vi "Sensor Indicator Map.vi"(8 "Action":T1, 10 "Control Lists In":refnum<vi>[][](array[refnum]), 11 "Sensor List In":T2[](array[typedef])) -> (2 "Control Lists Out":refnum<vi>[][](array[refnum]), 3 "Sensor List Out":T2[](array[typedef]))   [LabVIEW 2015]
uses:
  Sensor Enum.ctl
  Sensor Indicator Map Action.ctl
panel:
  in  "Sensor Enum":T2
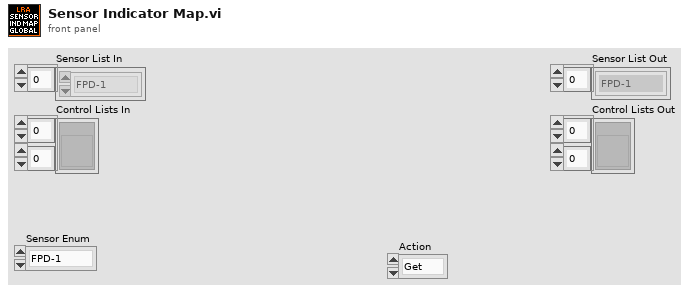
[diagram p1: front panel]
types:
  T1 = typedef "Sensor Indicator Map Action.ctl" = enum16{"Get", "Set"}
  T2 = typedef "Sensor Enum.ctl" = enum16{"FPD-1", "FPD-2", "FPD-3", "OPD-1", "OPD-2", "OPD-3", "AP-1", "VBAT", "VCOMP", "ICOMP", "TD10"}
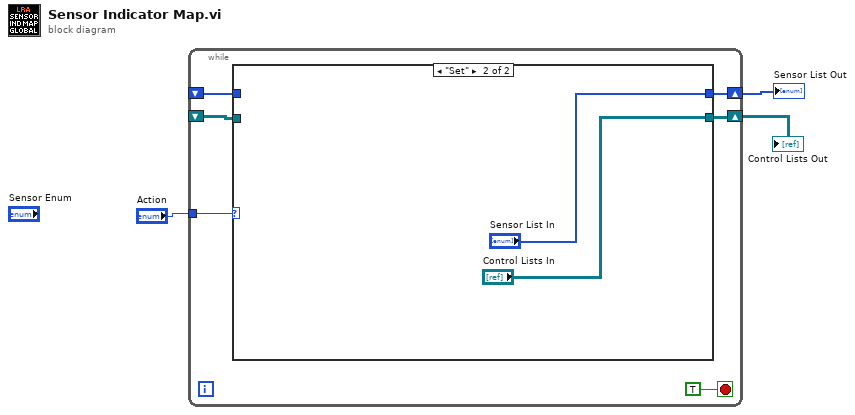
[diagram p0: block diagram]
diagram:
  n1 = while {
    shift-right: [w8] -> w3
    shift-left: _ -> [w4]
    tunnel: "Action" -> [w7]
    shift-right: [w6] -> w1
    shift-left: _ -> [w5]
    stop <- TRUE stop-if-true
    n2 = case shown="\"Set\"" w7 {
      tunnel: [w11 "Sensor List In"] -> w8
      tunnel: [w10 "Control Lists In"] -> w6
      tunnel: w5 -> [w10 _]
      tunnel: w4 -> [w11 _]
      frame "Get", Default {
      }
      frame "Set" {
      }
    }
  }
  "Sensor List Out" <- w3
  "Control Lists Out" <- w1
